vi "Write_VISA name.vi"(8 "error in (no error)":errorcluster, 10 "VISA resource name":refnum<visa-resource-name>, 11 "instrument in":refnum<class "instrument.lvclass">) -> (0 "error out":errorcluster, 3 "instrument out":refnum<class "instrument.lvclass">)   [LabVIEW 2018, in "instrument.lvclass"]
doc: "sets the \"VISA resource name\" of the object"
uses:
  instrument.lvclass
  instrument.lvclass/instrument.ctl
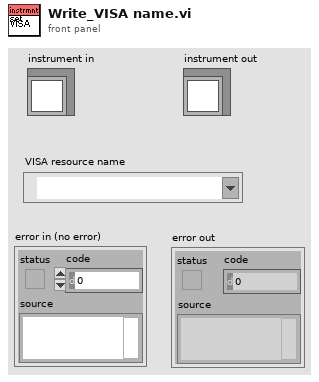
[diagram p1: front panel]
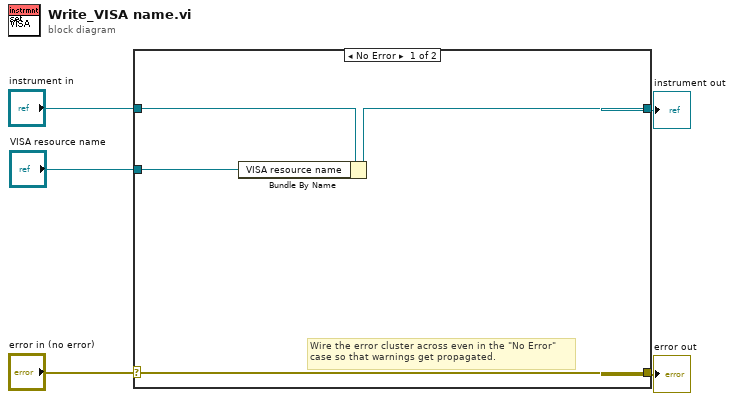
[diagram p0: block diagram]
diagram:
  n1 = case shown="No Error" "error in (no error)" {
    selector: "error in (no error)" -> [w9 w11]
    tunnel: [w9 w11] -> w4
    tunnel: [w7 w10] -> w2
    tunnel: "instrument in" -> [w8 w10]
    tunnel: "VISA resource name" -> [w6 _]
    frame No Error {
      # "Wire the error cluster across even in the \"No Error\"\ncase so that warnings get propagated."
      n2 = Bundle By Name(cluster=w8, "VISA resource name"=w6) -> (w7:refnum<class "instrument.lvclass">)
    }
    frame Error {
    }
  }
  "error out" <- w4
  "instrument out" <- w2
